vi "Find Clicked Decorations.vi"(10 "Coords":T1, 11 "Front Panel Objects":refnum<vi>[](array[refnum])) -> (3 "Found Decorations":string[](array[string]))   [LabVIEW 2019, in "LSS.lvlib"]
uses:
  LSS.lvlib
  <vilib>/Utility/miscctls.llb/LVPoint32TypeDef.ctl
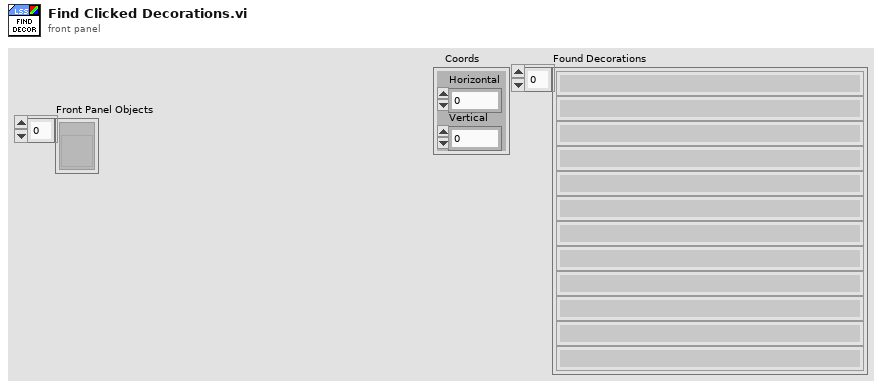
[diagram p1: front panel]
types:
  T1 = typedef "LVPoint32TypeDef.ctl" = cluster{"Horizontal":i32, "Vertical":i32}
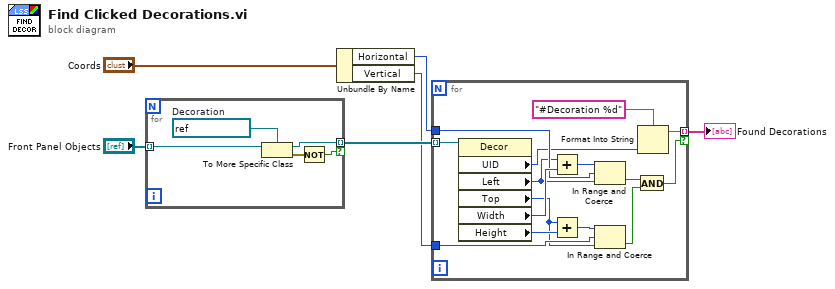
[diagram p0: block diagram]
diagram:
  n1 = for {
    tunnel: "Front Panel Objects" -> [w10] mode=indexing
    tunnel: [w9] -> w5 mode=indexing if=w7
    w11 = refnum<vi> refnum  # Decoration
    n2 = To More Specific Class(target class=w11, reference=w10) -> (specific class reference=w9:refnum<vi>, error out=w8:errorcluster)  [unwired: 1 in]
    n3 = Not(x=w8) -> (.not. x?=w7:bool)
  }
  n4 = Unbundle By Name("Coords") -> ("Horizontal"=w3:i32, "Vertical"=w2:i32)
  n5 = for {
    tunnel: w5 -> [w26] mode=indexing
    tunnel: w3 -> [w23]
    tunnel: w2 -> [w22]
    tunnel: [w16] -> w1 mode=indexing if=w19
    n6 = property class="Decor"(reference=w26) -> ("UID"=w17:i32, "Left"=w14:i32, "Top"=w12:i32, "Width"=w25:u32, "Height"=w24:u32)  [unwired: 1 in, 2 out]
    n7 = Add(x=w14, y=w25) -> (x+y=w15:u32)
    n8 = Add(x=w12, y=w24) -> (x+y=w13:u32)
    n9 = In Range and Coerce(upper limit=w15, x=w23, lower limit=w14) -> (In Range?=w21:bool)  [unwired: 1 out]
    n10 = In Range and Coerce(upper limit=w13, x=w22, lower limit=w12) -> (In Range?=w20:bool)  [unwired: 1 out]
    n11 = And(x=w21, y=w20) -> (x .and. y?=w19:bool)
    n12 = Format Into String(format string="#Decoration %d", w17) -> (resulting string=w16:string)  [unwired: 2 in, 1 out]
  }
  "Found Decorations" <- w1
